vi "BGP - Data - Temperature.vi"(8 "error in":errorcluster) -> (0 "error out":errorcluster)   [LabVIEW 2012]
uses:
  Controls/Object Ref and Name.ctl
  Controls/Global Stop States.ctl
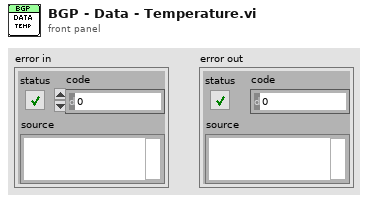
[diagram p1: front panel]
types:
  T1 = typedef "Object Ref and Name.ctl" = cluster{"Name":string, "Reference":refnum<vi>}
  T2 = typedef "Global Stop States.ctl" = enum16{"STOP", "STATUS", "INIT"}
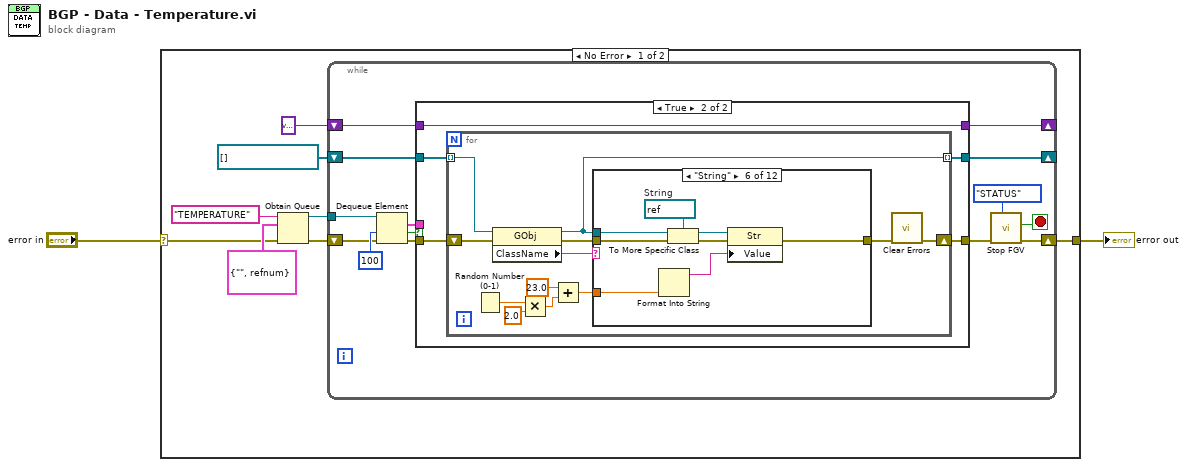
[diagram p0: block diagram]
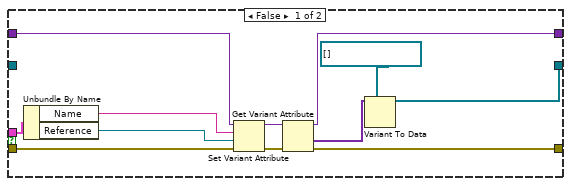
[diagram p2: hidden frame]
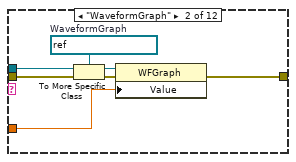
[diagram p4: hidden frame]
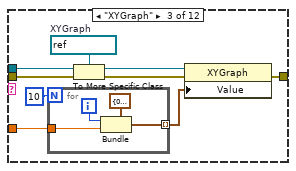
[diagram p5: hidden frame]
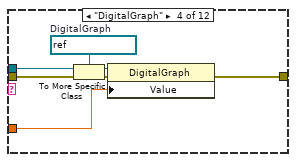
[diagram p6: hidden frame]
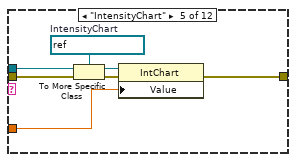
[diagram p7: hidden frame]
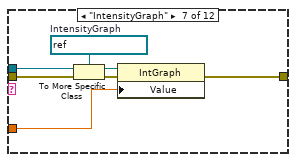
[diagram p8: hidden frame]
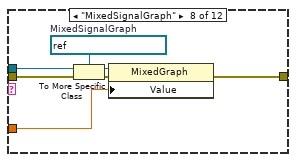
[diagram p9: hidden frame]
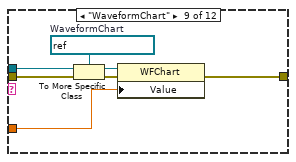
[diagram p10: hidden frame]
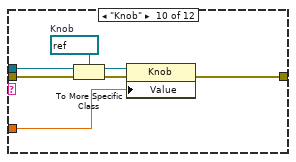
[diagram p11: hidden frame]
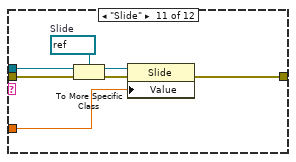
[diagram p12: hidden frame]
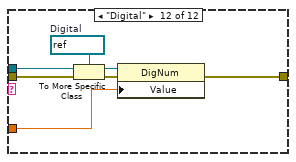
[diagram p13: hidden frame]
diagram:
  n1 = case shown="No Error" "error in" {
    selector: "error in" -> [w3 w139]
    tunnel: [w10 w139] -> w2
    frame No Error {
      n2 = Obtain Queue(name (unnamed)="TEMPERATURE", element data type=T1 {"Name"="", "Reference"=refnum}, error in (no error)=w3) -> (queue out=w4:refnum<queue>, error out=w8:errorcluster)  [unwired: 2 in, 1 out]
      n3 = while {
        tunnel: w4 -> [w24]
        shift-right: [w20] -> _
        shift-left: variant ("variant") -> [w22]
        shift-right: [w14] -> w10
        shift-left: w8 -> [w18]
        shift-right: [w17] -> _
        shift-left: refnum<vi>[] [] -> [w16]
        stop <- w11 stop-if-true
        n4 = Dequeue Element(queue=w24, timeout in ms (-1)=100, error in (no error)=w18) -> (element=w21:T1, timed out?=w15:bool, error out=w19:errorcluster)  [unwired: 1 out]
        n5 = case shown="True" w15 {
          tunnel: w22 -> [w36 w41]
          tunnel: w21 -> [w35 _]
          tunnel: [w31 w41] -> w20
          tunnel: w19 -> [w30 w40]
          tunnel: [w28 w37] -> w13
          tunnel: [w25 w38] -> w17
          tunnel: w16 -> [_ w39]
          frame False {
            n6 = Unbundle By Name(w35) -> ("Name"=w34:string, "Reference"=w33:refnum<vi>)
            n7 = Set Variant Attribute(Variant=w36, name=w34, value=w33, error in=w30) -> (Variant out=w32:variant, error out=w29:errorcluster)  [unwired: 1 out]
            n8 = Get Variant Attribute(Variant=w32, error in=w29) -> (duplicate Variant=w31:variant, values=w26:variant[], error out=w28:errorcluster)  [unwired: 2 in, 1 out]
            n9 = Variant To Data(type=refnum<vi>[] [], Variant=w26) -> (data=w25:refnum<vi>[])  [unwired: 1 in, 1 out]
          }
          frame True {
            n10 = for {
              tunnel: w39 -> [w49] mode=indexing
              shift-right: [w45] -> w37
              shift-left: w40 -> [w47]
              tunnel: [w48] -> w38 mode=indexing
              n11 = Random Number (0-1)() -> (number: 0 to 1=w53:dbl)
              n12 = property class="GObj"(reference=w49, error in=w47) -> (reference out=w48:refnum<vi>, error out=w46:errorcluster, "ClassName"=w43:string)
              n13 = Multiply(x=w53, y=2.0) -> (x*y=w42:dbl)
              n14 = Add(x=23.0 ("y"), y=w42) -> (x+y=w50:dbl)
              n15 = case shown="\"String\"" w43 {
                tunnel: w50 -> [_ w59 w62 w79 w86 w90 w101 w108 w115 w122 w129 w136]
                tunnel: w48 -> [_ w58 w68 w78 w85 w92 w100 w107 w114 w121 w128 w135]
                tunnel: w46 -> [w54 w56 w66 w76 w83 w91 w98 w105 w112 w119 w126 w133]
                tunnel: [w54 w57 w67 w77 w84 w89 w99 w106 w113 w120 w127 w134] -> w44
                frame "False", Default {
                }
                frame "WaveformGraph" {
                  w61 = refnum<vi> refnum  # WaveformGraph
                  n16 = To More Specific Class(target class=w61, reference=w58, error in=w56) -> (specific class reference=w60:refnum<vi>, error out=w55:errorcluster)
                  n17 = property class="WFGraph"(reference=w60, error in=w55, "Value"=w59) -> (error out=w57:errorcluster)  [unwired: 1 out]
                }
                frame "XYGraph" {
                  w70 = refnum<vi> refnum  # XYGraph
                  n18 = for {
                    N: 10 -> [_]
                    tunnel: [w73] -> w63 mode=indexing
                    tunnel: w62 -> [w71]
                    i -> [w72]
                    n19 = Bundle(cluster=cluster{dbl, dbl} {0.0, 0.0}, w72, w71) -> (w73:cluster{dbl, dbl})
                  }
                  n20 = To More Specific Class(target class=w70, reference=w68, error in=w66) -> (specific class reference=w69:refnum<vi>, error out=w65:errorcluster)
                  n21 = property class="XYGraph"(reference=w69, error in=w65, "Value"=w63) -> (error out=w67:errorcluster)  [unwired: 1 out]
                }
                frame "DigitalGraph" {
                  w81 = refnum<vi> refnum  # DigitalGraph
                  n22 = To More Specific Class(target class=w81, reference=w78, error in=w76) -> (specific class reference=w80:refnum<vi>, error out=w75:errorcluster)
                  n23 = property class="DigitalGraph"(reference=w80, error in=w75, "Value"=w79) -> (error out=w77:errorcluster)  [unwired: 1 out]
                }
                frame "IntensityChart" {
                  w88 = refnum<vi> refnum  # IntensityChart
                  n24 = To More Specific Class(target class=w88, reference=w85, error in=w83) -> (specific class reference=w87:refnum<vi>, error out=w82:errorcluster)
                  n25 = property class="IntChart"(reference=w87, error in=w82, "Value"=w86) -> (error out=w84:errorcluster)  [unwired: 1 out]
                }
                frame "String" {
                  w93 = refnum<vi> refnum  # String
                  n26 = Format Into String(w90) -> (resulting string=w96:string)  [unwired: 3 in, 1 out]
                  n27 = To More Specific Class(target class=w93, reference=w92, error in=w91) -> (specific class reference=w94:refnum<vi>, error out=w95:errorcluster)
                  n28 = property class="Str"(reference=w94, error in=w95, "Value"=w96) -> (error out=w89:errorcluster)  [unwired: 1 out]
                }
                frame "IntensityGraph" {
                  w103 = refnum<vi> refnum  # IntensityGraph
                  n29 = To More Specific Class(target class=w103, reference=w100, error in=w98) -> (specific class reference=w102:refnum<vi>, error out=w97:errorcluster)
                  n30 = property class="IntGraph"(reference=w102, error in=w97, "Value"=w101) -> (error out=w99:errorcluster)  [unwired: 1 out]
                }
                frame "MixedSignalGraph" {
                  w110 = refnum<vi> refnum  # MixedSignalGraph
                  n31 = To More Specific Class(target class=w110, reference=w107, error in=w105) -> (specific class reference=w109:refnum<vi>, error out=w104:errorcluster)
                  n32 = property class="MixedGraph"(reference=w109, error in=w104, "Value"=w108) -> (error out=w106:errorcluster)  [unwired: 1 out]
                }
                frame "WaveformChart" {
                  w117 = refnum<vi> refnum  # WaveformChart
                  n33 = To More Specific Class(target class=w117, reference=w114, error in=w112) -> (specific class reference=w116:refnum<vi>, error out=w111:errorcluster)
                  n34 = property class="WFChart"(reference=w116, error in=w111, "Value"=w115) -> (error out=w113:errorcluster)  [unwired: 1 out]
                }
                frame "Knob" {
                  w124 = refnum<vi> refnum  # Knob
                  n35 = To More Specific Class(target class=w124, reference=w121, error in=w119) -> (specific class reference=w123:refnum<vi>, error out=w118:errorcluster)
                  n36 = property class="Knob"(reference=w123, error in=w118, "Value"=w122) -> (error out=w120:errorcluster)  [unwired: 1 out]
                }
                frame "Slide" {
                  w131 = refnum<vi> refnum  # Slide
                  n37 = To More Specific Class(target class=w131, reference=w128, error in=w126) -> (specific class reference=w130:refnum<vi>, error out=w125:errorcluster)
                  n38 = property class="Slide"(reference=w130, error in=w125, "Value"=w129) -> (error out=w127:errorcluster)  [unwired: 1 out]
                }
                frame "Digital" {
                  w138 = refnum<vi> refnum  # Digital
                  n39 = To More Specific Class(target class=w138, reference=w135, error in=w133) -> (specific class reference=w137:refnum<vi>, error out=w132:errorcluster)
                  n40 = property class="DigNum"(reference=w137, error in=w132, "Value"=w136) -> (error out=w134:errorcluster)  [unwired: 1 out]
                }
              }
              n41 = call <vilib>:"Clear Errors.vi"("error in (no error)"=w44) -> ("error out"=w45:errorcluster)  [unwired: 6 in]
            }
          }
        }
        n42 = call "Stop FGV.vi"("Operation In"=Global_Stop_States."STATUS", "error in"=w13) -> ("error out"=w14:errorcluster, "Stop?"=w11:bool)  [unwired: 8 in]
      }
    }
    frame Error {
    }
  }
  "error out" <- w2
